vi "停止整机测试(子VI).vi"() -> (0 "error out":T1={"status"=FALSE, "代码"=4, "source"=""} caption="错误输出" {"代码" items=["执行成功"=1, "执行失败，但不知道原因"=2, "命令请求条件错误"=3, "通讯超时"=4, "系统繁忙不能执行"=5, "系统故障"=6, "没有数据"=100]})   [LabVIEW 2016]
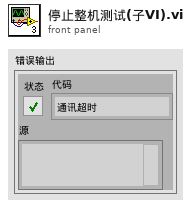
[diagram p1: front panel]
types:
  T1 = cluster{"status":bool, "代码":u16, "source":string}
  T2 = cluster{"命令":string, cluster{"starting address":u16, "holding register value":u16}}
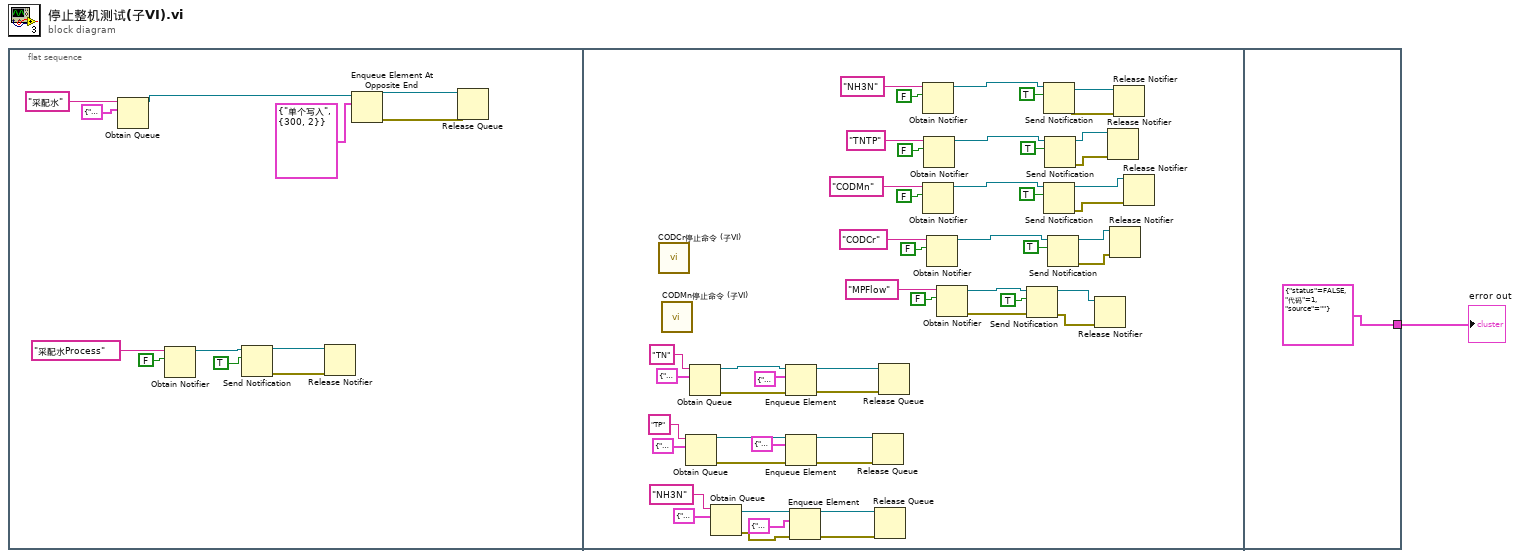
[diagram p0: block diagram]
diagram:
  n1 = flat-sequence {
    tunnel: [T1 {"status"=FALSE, "代码"=1, "source"=""} ("error out")] -> w1
    frame #0 {
      n2 = Obtain Queue(name (unnamed)="采配水" ("名称（未命名）"), element data type=cluster{"命令":string, "数据":variant} {"命令"="", "数据"=variant}) -> (queue out=w11:refnum<queue>)  [unwired: 3 in, 2 out]
      n3 = Obtain Notifier(name (unnamed)="采配水Process" ("名称（未命名）"), notification data type=FALSE) -> (notifier out=w13:refnum<notifier>)  [unwired: 2 in, 2 out]
      n4 = Send Notification(notification=TRUE ("通知"), notifier=w13) -> (notifier out=w3:refnum<notifier>, error out=w2:errorcluster)  [unwired: 1 in]
      n5 = Release Notifier(notifier=w3, error in (no error)=w2) -> ()  [unwired: 1 in, 3 out]
      n6 = Enqueue Element At Opposite End(queue=w11, element=T2 {"命令"="单个写入", {"starting address"=300, "holding register value"=2}} ("元素")) -> (queue out=w5:refnum<queue>, error out=w4:errorcluster)  [unwired: 2 in, 1 out]
      n7 = Release Queue(queue=w5, error in (no error)=w4) -> ()  [unwired: 1 in, 3 out]
    }
    frame #1 {
      n8 = call "CODCr停止命令 (子VI).vi"() -> ()  [unwired: 12 in]
      n9 = call "CODMn停止命令 (子VI).vi"() -> ()  [unwired: 12 in]
      n10 = Obtain Queue(name (unnamed)="TP" ("名称（未命名）"), element data type=cluster{"命令":string, "data":variant} {"命令"="", "data"=variant}) -> (queue out=w58:refnum<queue>, error out=w35:errorcluster)  [unwired: 3 in, 1 out]
      n11 = Obtain Queue(name (unnamed)="TN" ("名称（未命名）"), element data type=cluster{"命令":string, "data":variant} {"命令"="", "data"=variant}) -> (queue out=w31:refnum<queue>, error out=w30:errorcluster)  [unwired: 3 in, 1 out]
      n12 = Obtain Queue(name (unnamed)="NH3N" ("名称（未命名）"), element data type=cluster{"命令":string, "data":variant} {"命令"="", "data"=variant}) -> (queue out=w65:refnum<queue>, error out=w34:errorcluster)  [unwired: 3 in, 1 out]
      n13 = Enqueue Element(queue=w31, element=cluster{"命令":string, "data":variant} {"命令"="启动", "data"=variant(cluster{"站号":u16, "控制命令输出":u16[]} {"站号"=2, "控制命令输出"=[2816]})} ("元素"), error in (no error)=w30) -> (queue out=w29:refnum<queue>, error out=w28:errorcluster)  [unwired: 1 in, 1 out]
      n14 = Enqueue Element(queue=w58, element=cluster{"命令":string, "data":variant} {"命令"="启动", "data"=variant(cluster{"站号":u16, "控制命令输出":u16[]} {"站号"=1, "控制命令输出"=[2816]})} ("元素"), error in (no error)=w35) -> (queue out=w27:refnum<queue>, error out=w26:errorcluster)  [unwired: 1 in, 1 out]
      n15 = Enqueue Element(queue=w65, element=cluster{"命令":string, "data":variant} {"命令"="启动", "data"=variant(cluster{"站号":u16, "控制命令输出":u16[]} {"站号"=3, "控制命令输出"=[2816]})} ("启动命令"), error in (no error)=w34) -> (queue out=w25:refnum<queue>, error out=w24:errorcluster)  [unwired: 1 in, 1 out]
      n16 = Release Queue(queue=w27, error in (no error)=w26) -> ()  [unwired: 1 in, 3 out]
      n17 = Release Queue(queue=w25, error in (no error)=w24) -> ()  [unwired: 1 in, 3 out]
      n18 = Release Queue(queue=w29, error in (no error)=w28) -> ()  [unwired: 1 in, 3 out]
      n19 = Obtain Notifier(name (unnamed)="NH3N" ("名称（未命名）"), notification data type=FALSE) -> (notifier out=w62:refnum<notifier>)  [unwired: 2 in, 2 out]
      n20 = Obtain Notifier(name (unnamed)="CODMn" ("名称（未命名）"), notification data type=FALSE) -> (notifier out=w47:refnum<notifier>)  [unwired: 2 in, 2 out]
      n21 = Obtain Notifier(name (unnamed)="TNTP" ("名称（未命名）"), notification data type=FALSE) -> (notifier out=w54:refnum<notifier>)  [unwired: 2 in, 2 out]
      n22 = Obtain Notifier(name (unnamed)="CODCr" ("名称（未命名）"), notification data type=FALSE) -> (notifier out=w41:refnum<notifier>)  [unwired: 2 in, 2 out]
      n23 = Obtain Notifier(name (unnamed)="MPFlow" ("名称（未命名）"), notification data type=FALSE) -> (notifier out=w43:refnum<notifier>, error out=w42:errorcluster)  [unwired: 2 in, 1 out]
      n24 = Send Notification(notification=TRUE ("通知"), notifier=w43, error in (no error)=w42) -> (notifier out=w15:refnum<notifier>, error out=w14:errorcluster)
      n25 = Send Notification(notification=TRUE ("通知"), notifier=w62) -> (notifier out=w23:refnum<notifier>, error out=w22:errorcluster)  [unwired: 1 in]
      n26 = Send Notification(notification=TRUE ("通知"), notifier=w47) -> (notifier out=w19:refnum<notifier>, error out=w18:errorcluster)  [unwired: 1 in]
      n27 = Send Notification(notification=TRUE ("通知"), notifier=w54) -> (notifier out=w21:refnum<notifier>, error out=w20:errorcluster)  [unwired: 1 in]
      n28 = Send Notification(notification=TRUE ("通知"), notifier=w41) -> (notifier out=w17:refnum<notifier>, error out=w16:errorcluster)  [unwired: 1 in]
      n29 = Release Notifier(notifier=w15, error in (no error)=w14) -> ()  [unwired: 1 in, 3 out]
      n30 = Release Notifier(notifier=w21, error in (no error)=w20) -> ()  [unwired: 1 in, 3 out]
      n31 = Release Notifier(notifier=w17, error in (no error)=w16) -> ()  [unwired: 1 in, 3 out]
      n32 = Release Notifier(notifier=w23, error in (no error)=w22) -> ()  [unwired: 1 in, 3 out]
      n33 = Release Notifier(notifier=w19, error in (no error)=w18) -> ()  [unwired: 1 in, 3 out]
    }
    frame #2 {
    }
  }
  "error out" <- w1
